vi "Send Read Sink Settings.vi"(7 "Priority":T1=enum."Normal" caption="Message Priority (Normal)", 8 "error in (no error)":errorcluster, 10 "Sink Name":string, 11 "Message Enqueuer in":refnum<class "Message Enqueuer.lvclass">) -> (0 "error out":errorcluster, 3 "Message Enqueuer out":refnum<class "Message Enqueuer.lvclass">)   [LabVIEW 2016, in "Event Source.lvlib" / "Read Sink Settings Msg.lvclass"]
doc: "Sends the <b>Event Source.lvlib:Read Sink Settings Msg.lvclass</b> message.\n\nThis message will call <b>Read Sink Settings.vi</b> on the <b>Event Source.lvlib:Event Source.lvclass</b> actor.\n\n<b>Read Sink Settings.vi Description</b>\nAllows to set the Sink behaviour by setting the following flags\n\n\"Exclude From Broadcast\"\nmessage originating form another sink will not be broadcasted to the sink being cosidered\n\"Paused\"\nThe sink will not send events and will not receive them anymore\n\"Receive only\"\nThe sing will receive events but not sany any"
uses:
  Read Sink Settings Msg.lvclass
  <vilib>/ActorFramework/Message Enqueuer/Message Enqueuer.lvclass
  <vilib>/ActorFramework/Message Enqueuer/Message Priority.ctl
  C:/Program Files (x86)/National Instruments/LabVIEW 2016/vi.lib/ActorFramework/Message/Message.lvclass
  Read Sink Settings Msg.lvclass/Read Sink Settings Msg.ctl
  <vilib>/ActorFramework/Message Enqueuer/Message Enqueuer.lvclass/Message Enqueuer.ctl
  <vilib>/Utility/LVClass/Get LV Class Name.vi
  <resource>/AFDebug/Generate Trace for Message.vi
  <vilib>/ActorFramework/Message Priority Queue/Priority Enqueue.vi
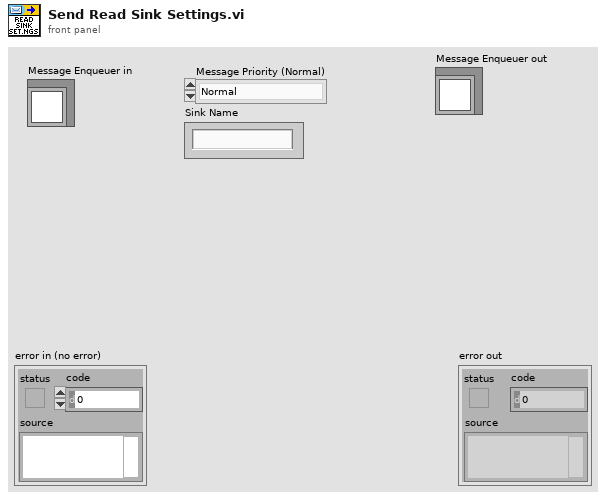
[diagram p1: front panel]
types:
  T1 = typedef "Actor Framework.lvlib/Message Enqueuer.lvclass/Message Priority.ctl" = enum16{"Low", "Normal", "High"}
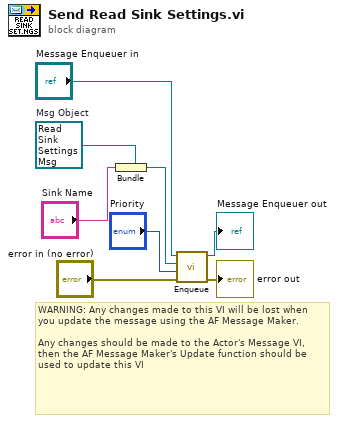
[diagram p0: block diagram]
diagram:
  w7 = refnum<class "Read Sink Settings Msg.lvclass"> refnum  # Msg Object
  # "WARNING: Any changes made to this VI will be lost when you update the message using the AF Message Maker.\n\nAny changes should be made to the Actor's Message VI, then the AF Message Maker's Update function should be used to update this VI"
  n1 = Bundle(cluster=w7, "Sink Name") -> (w2:refnum<class "Read Sink Settings Msg.lvclass">)
  n2 = call <vilib>:"Enqueue.vi"("error in (no error)"="error in (no error)", "Message Priority (Normal)"="Priority", "Message"=w2, "Message Enqueuer in"="Message Enqueuer in") -> ("error out"=→"error out":errorcluster, "Message Enqueuer out"=→"Message Enqueuer out":refnum<class "Message Enqueuer.lvclass">)  [unwired: 6 in]
